vi "Joystick and Camera SHIH V4- external Connection.vi"(0 "Motion in":refnum<class "Motion.lvclass">, 1 "XYZTheta":dbl[](array[numeric])=[584.964, 676.042, 69.3079, 0.000384], 2 "Measurement Point":string, 3 "Inital GO":bool=TRUE) -> (5 "final out":dbl[](array[numeric]), 7 "Motion out":refnum<class "Motion.lvclass">, 10 "error out":errorcluster)   [LabVIEW 2016]
uses:
  Classes/Controllers/Motion/Copy of Motion Folder/Motion.lvclass
panel:
  out "Gantry position":dbl[](array[numeric])
  in  "start measurement":bool
  in  "Joystick":bool
  in  "Stop":bool
  # "new world"
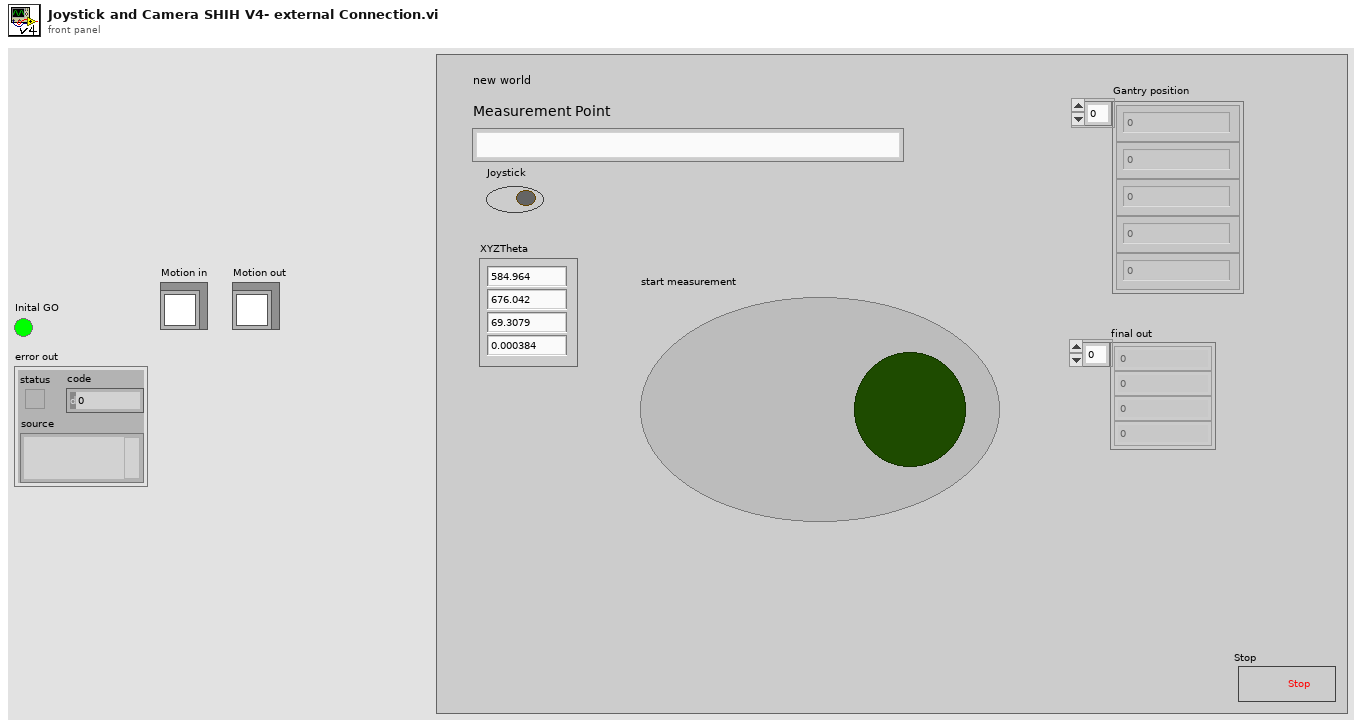
[diagram p1: front panel]
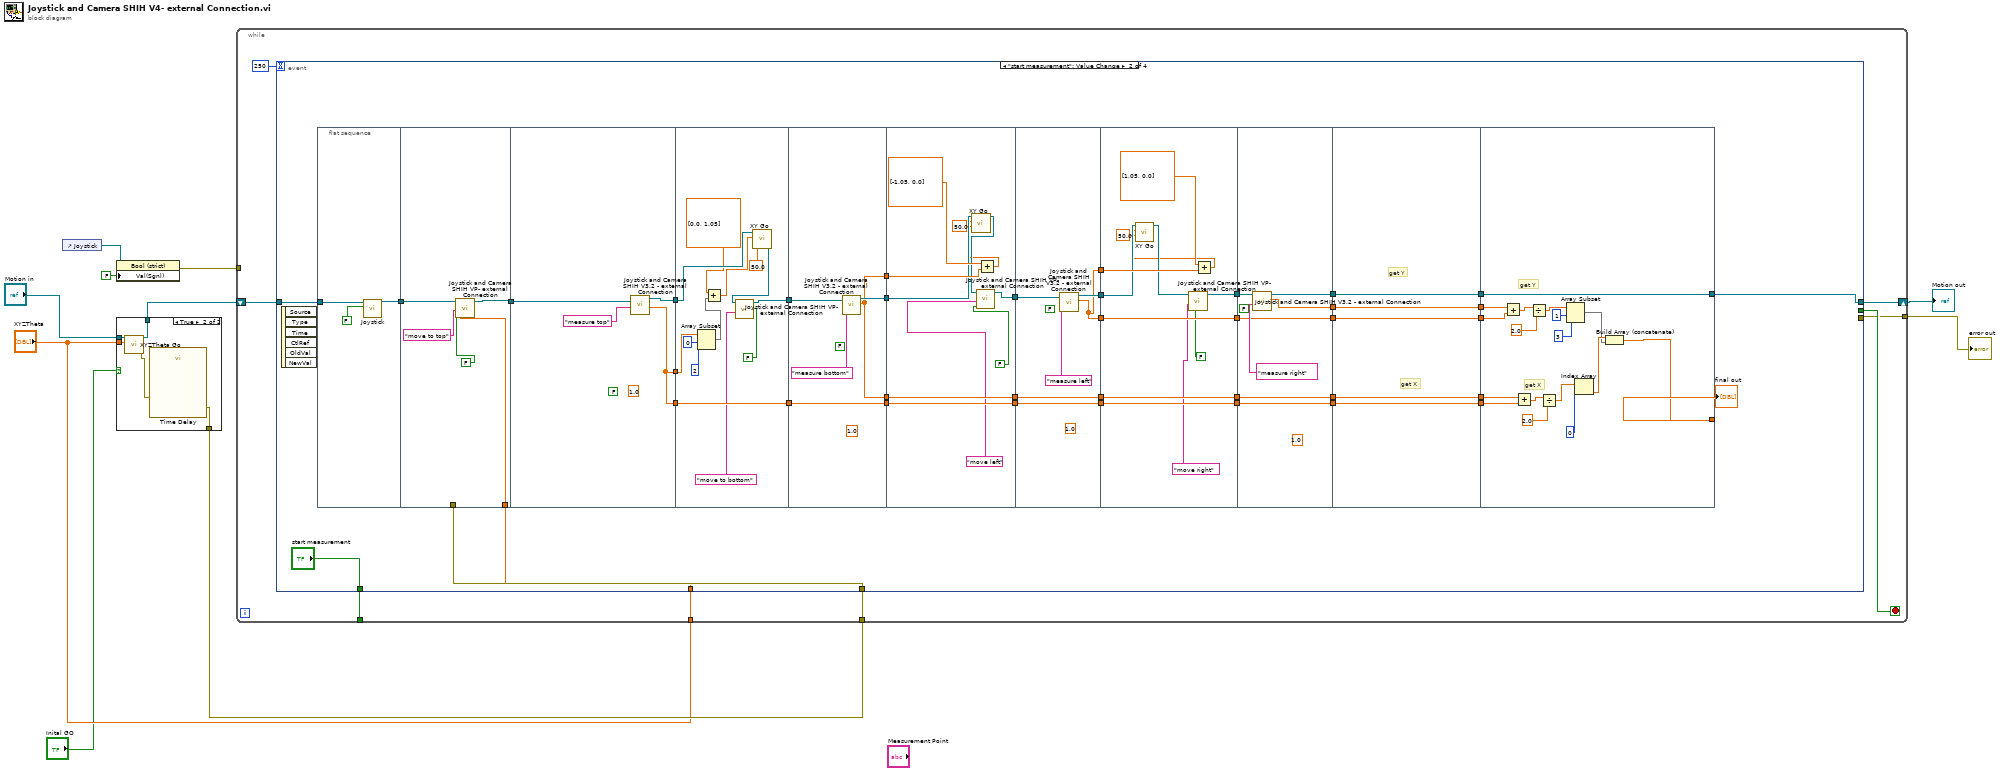
[diagram p0: block diagram]
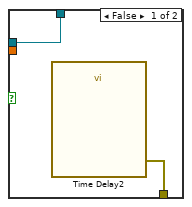
[diagram p2: hidden frame]
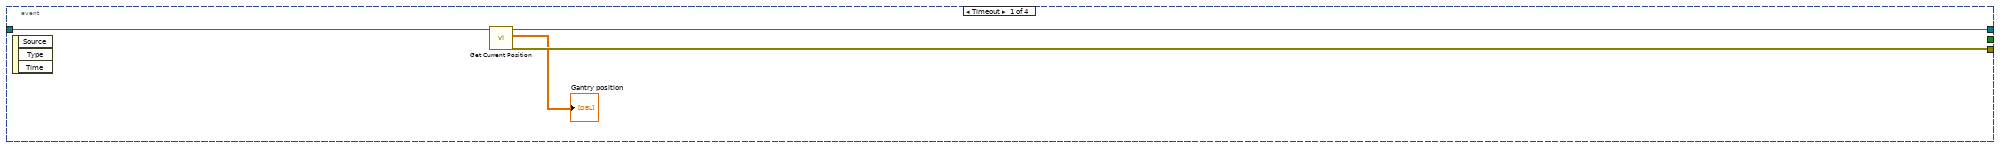
[diagram p3: hidden frame]
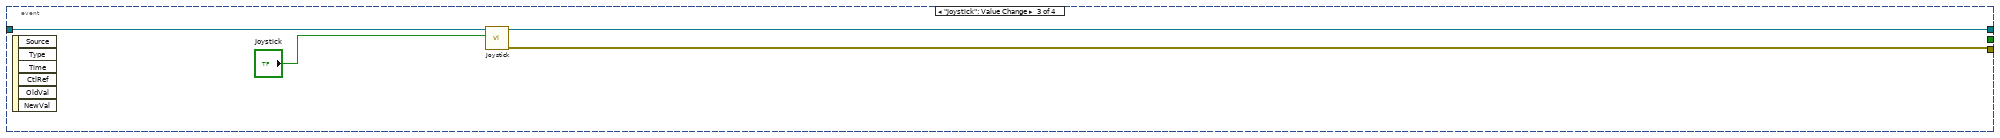
[diagram p4: hidden frame]
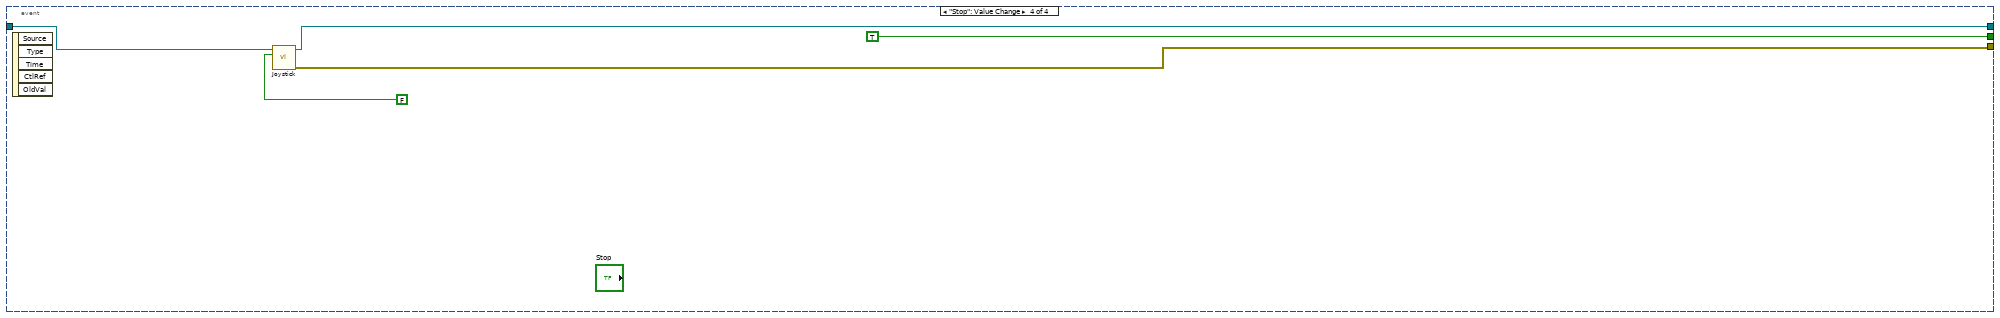
[diagram p5: hidden frame]
diagram:
  n1 = control-ref of="Joystick"() -> (w9:refnum<vi>)
  n2 = case shown="True" "Inital GO" {
    tunnel: "Motion in" -> [w12 w17]
    tunnel: [w12 w16] -> w4
    tunnel: [w11 w14] -> w3
    tunnel: "XYZTheta" -> [_ w13]
    frame False {
      n3 = call "Time Delay2"() -> ("error out"=w11:errorcluster)  [unwired: 11 in]
    }
    frame True {
      n4 = call "XYZTheta Go.vi"("XYZTheta In"=w13, "Motion in"=w17) -> ("error out"=w15:errorcluster, "Motion out"=w16:refnum<class "Motion.lvclass">)  [unwired: 7 in, 1 out]
      n5 = call "Time Delay"("error in (no error)"=w15) -> ("error out"=w14:errorcluster)  [unwired: 10 in]
    }
  }
  n6 = property class="Bool (strict)"(reference=w9, "Val(Sgnl)"=FALSE ("Value (Signaling)")) -> (error out=w8:errorcluster)  [unwired: 1 in, 1 out]
  n7 = while {
    shift-right: [w22] -> w7
    shift-left: w4 -> [w23]
    tunnel: w8 -> [_]
    tunnel: [w21] -> w6
    tunnel: w3 -> [w20]
    tunnel: "XYZTheta" -> [w19]
    tunnel: [w18] -> _
    stop <- w24 stop-if-true
    n8 = event shown="[1] \"start measurement\": Value Change" {
      selector: _ -> [_ _ _ _]
      dyn-events: _ -> [_ _ _ _]
      timeout: 250 -> [_ _ _ _]
      tunnel: [_ _ _ TRUE] -> w24
      tunnel: w23 -> [w29 w68 w160 w164]
      tunnel: [w28 w43 w158 w163] -> w22
      tunnel: [w27 _ w157 w161] -> w21
      tunnel: w20 -> [_ w67 _ _]
      tunnel: w19 -> [_ w45 _ _]
      tunnel: [_ "start measurement" _ _] -> w18
      event Timeout {
        n9 = event-data() -> ()  [unwired: 1 in, 3 out]
        n10 = call-dynamic "Get Current Position.vi"("Motion in"=w29) -> ("error out"=w27:errorcluster, "XYZTheta Out"=→"Gantry position":dbl[], "Motion out"=w28:refnum<class "Motion.lvclass">)  [unwired: 8 in]
      }
      event "start measurement": Value Change {
        n11 = event-data() -> ()  [unwired: 1 in, 6 out]
        n12 = flat-sequence {
          tunnel: w68 -> [w70]
          tunnel: [w69] -> w65
          tunnel: w67 -> [_]
          tunnel: [w72] -> w66
          tunnel: w65 -> [w76]
          tunnel: w45 -> [w73]
          tunnel: w66 -> [w80]
          tunnel: [w79] -> w64
          tunnel: [w77] -> w53
          tunnel: [w77] -> w42
          tunnel: w64 -> [w89]
          tunnel: [w92] -> w63
          tunnel: [w93] -> w54
          tunnel: w53 -> [w93]
          tunnel: w42 -> [w84]
          tunnel: w63 -> [w98]
          tunnel: [w96] -> w62
          tunnel: [w95] -> w55
          tunnel: w54 -> [w95]
          tunnel: [w94] -> w49
          tunnel: [w94] -> w41
          tunnel: w62 -> [w102]
          tunnel: [w107] -> w61
          tunnel: [w109] -> w56
          tunnel: w55 -> [w109]
          tunnel: [w108] -> w50
          tunnel: w49 -> [w108]
          tunnel: w41 -> [w103]
          tunnel: w61 -> [w115]
          tunnel: [w114] -> w60
          tunnel: [w112] -> w57
          tunnel: w56 -> [w112]
          tunnel: [w111] -> w51
          tunnel: w50 -> [w111]
          tunnel: [w110] -> w47
          tunnel: [w110] -> w40
          tunnel: w60 -> [w119]
          tunnel: [w124] -> w59
          tunnel: [w127] -> w58
          tunnel: w57 -> [w127]
          tunnel: [w126] -> w52
          tunnel: w51 -> [w126]
          tunnel: [w125] -> w48
          tunnel: w47 -> [w125]
          tunnel: w40 -> [w120]
          tunnel: w59 -> [w134]
          tunnel: [w132] -> w39
          tunnel: w58 -> [w132]
          tunnel: [w131] -> w37
          tunnel: w52 -> [w131]
          tunnel: [w130] -> w35
          tunnel: [w129] -> w33
          tunnel: w48 -> [w129]
          tunnel: [w128] -> w31
          tunnel: w39 -> [w139]
          tunnel: [w139] -> w38
          tunnel: w37 -> [w138]
          tunnel: [w138] -> w36
          tunnel: w35 -> [w137]
          tunnel: [w137] -> w34
          tunnel: w33 -> [w136]
          tunnel: [w136] -> w32
          tunnel: w31 -> [w135]
          tunnel: [w135] -> w30
          tunnel: w38 -> [w156]
          tunnel: w36 -> [w155]
          tunnel: w34 -> [w150]
          tunnel: w32 -> [w149]
          tunnel: [w141] -> w44
          tunnel: w30 -> [w140]
          tunnel: [w140] -> w43
          frame #0 {
            n13 = call-dynamic "Joystick.vi"("Joystick"=FALSE, "Motion in"=w70) -> ("Motion out"=w69:refnum<class "Motion.lvclass">)  [unwired: 8 in, 1 out]
          }
          frame #1 {
            n14 = call "Joystick and Camera SHIH VP- external Connection.vi"("Motion in"=w76, "XYZTheta"=w73, "Measurement Point"="move to top", "Inital GO"=FALSE) -> ("Motion out"=w72:refnum<class "Motion.lvclass">)  [unwired: 3 in, 3 out]
          }
          frame #2 {
            (unwired) 1.0 ("reset the counting")
            (unwired) FALSE ("Inital GO")
            n15 = call "Joystick and Camera SHIH V3.2 - external Connection.vi"("Measurement Point"="measure top", "Motion in"=w80) -> ("final out"=w77:dbl[], "Motion out 2"=w79:refnum<class "Motion.lvclass">)  [unwired: 3 in, 3 out]
          }
          frame #3 {
            n16 = Array Subset(array=w84, index=0, length=2) -> (w82:dbl[])
            n17 = Add(x=dbl[] [0.0, 1.05], y=w82) -> (x+y=w81:dbl[])
            n18 = call-dynamic "XY Go.vi"("Speed"=50.0, "XY"=w81, "Motion in"=w89) -> ("Motion out"=w88:refnum<class "Motion.lvclass">)  [unwired: 7 in, 1 out]
            n19 = call "Joystick and Camera SHIH VP- external Connection.vi"("Motion in"=w88, "Measurement Point"="move to bottom", "Inital GO"=FALSE) -> ("Motion out"=w92:refnum<class "Motion.lvclass">)  [unwired: 4 in, 3 out]
          }
          frame #4 {
            (unwired) 1.0 ("reset the counting")
            (unwired) FALSE ("Inital GO")
            n20 = call "Joystick and Camera SHIH V3.2 - external Connection.vi"("Measurement Point"="measure bottom", "Motion in"=w98) -> ("final out"=w94:dbl[], "Motion out 2"=w96:refnum<class "Motion.lvclass">)  [unwired: 3 in, 3 out]
          }
          frame #5 {
            n21 = Add(x=dbl[] [-1.05, 0.0], y=w103) -> (x+y=w100:dbl[])
            n22 = call-dynamic "XY Go.vi"("Speed"=50.0, "XY"=w100, "Motion in"=w102) -> ("Motion out"=w101:refnum<class "Motion.lvclass">)  [unwired: 7 in, 1 out]
            n23 = call "Joystick and Camera SHIH VP- external Connection.vi"("Motion in"=w101, "Measurement Point"="move left", "Inital GO"=FALSE) -> ("Motion out"=w107:refnum<class "Motion.lvclass">)  [unwired: 4 in, 3 out]
          }
          frame #6 {
            (unwired) 1.0 ("reset the counting")
            (unwired) FALSE ("Inital GO")
            n24 = call "Joystick and Camera SHIH V3.2 - external Connection.vi"("Measurement Point"="measure left", "Motion in"=w115) -> ("final out"=w110:dbl[], "Motion out 2"=w114:refnum<class "Motion.lvclass">)  [unwired: 3 in, 3 out]
          }
          frame #7 {
            n25 = Add(x=dbl[] [1.05, 0.0], y=w120) -> (x+y=w117:dbl[])
            n26 = call-dynamic "XY Go.vi"("Speed"=50.0, "XY"=w117, "Motion in"=w119) -> ("Motion out"=w118:refnum<class "Motion.lvclass">)  [unwired: 7 in, 1 out]
            n27 = call "Joystick and Camera SHIH VP- external Connection.vi"("Motion in"=w118, "Measurement Point"="move right", "Inital GO"=FALSE) -> ("Motion out"=w124:refnum<class "Motion.lvclass">)  [unwired: 4 in, 3 out]
          }
          frame #8 {
            (unwired) 1.0 ("reset the counting")
            (unwired) FALSE ("Inital GO")
            n28 = call "Joystick and Camera SHIH V3.2 - external Connection.vi"("Measurement Point"="measure right", "Motion in"=w134) -> ("final out"=w130:dbl[], "Motion out 2"=w128:refnum<class "Motion.lvclass">)  [unwired: 3 in, 3 out]
          }
          frame #9 {
            # "get X"
            # "get Y"
          }
          frame #10 {
            # "get X"
            # "get Y"
            n29 = Add(x=w150, y=w149) -> (x+y=w151:dbl[])
            n30 = Add(x=w155, y=w156) -> (x+y=w153:dbl[])
            n31 = Divide(x=w151, y=2.0) -> (x/y=w146:dbl[])
            n32 = Divide(x=w153, y=2.0) -> (x/y=w148:dbl[])
            n33 = Array Subset(array=w146, index=1, length=3) -> (w142:dbl[])
            n34 = Index Array(array=w148, index=0) -> (element=w143:dbl)
            n35 = Build Array (concatenate)(w143, w142) -> (w141:dbl[])
          }
        }
        "final out" <- w44
      }
      event "Joystick": Value Change {
        n36 = event-data() -> ()  [unwired: 1 in, 6 out]
        n37 = call-dynamic "Joystick.vi"("Joystick"="Joystick", "Motion in"=w160) -> ("error out"=w157:errorcluster, "Motion out"=w158:refnum<class "Motion.lvclass">)  [unwired: 8 in]
      }
      event "Stop": Value Change {
        n38 = event-data() -> ()  [unwired: 1 in, 5 out]
        n39 = call-dynamic "Joystick.vi"("Joystick"=FALSE, "Motion in"=w164) -> ("error out"=w161:errorcluster, "Motion out"=w163:refnum<class "Motion.lvclass">)  [unwired: 8 in]
      }
    }
  }
  "error out" <- w6
  "Motion out" <- w7
